vi "计时.vi"(2 "s":bool, 3 "y":i64) -> (1 "x-y":i64)   [LabVIEW 2012]
panel:
  out "s? t:f":i64
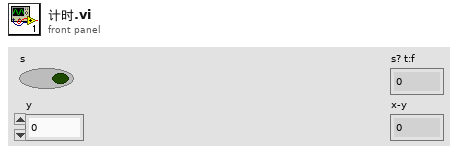
[diagram p1: front panel]
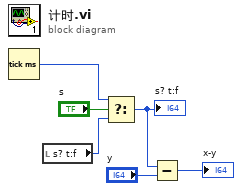
[diagram p0: block diagram]
diagram:
  n1 = Tick Count (ms)() -> (millisecond timer value=w5:u32)
  n2 = local read "s? t:f"() -> (w4:i64)
  n3 = Select(t=w5, s="s", f=w4) -> (s? t:f=w3:i64)
  "s? t:f" <- w3
  n4 = Subtract(x=w3, y="y") -> (x-y=→"x-y":i64)
